vi "FPGA_PPG_VI_Tree.vi"   [LabVIEW 2014, in "NI-FPGA_PPG_Driver.lvlib"]
doc: "This is a VI tree containing all VIs that are available to the user.\n\nDietrich Beck, GSI Helmholtzzentrum fuer Schwerionenforschung, Germany\noriginal author: Falk Ziegler, Falk Ziegler, ziegler@physik.uni-greifswald.de"
uses:
  NI-FPGA_PPG_Driver.lvlib
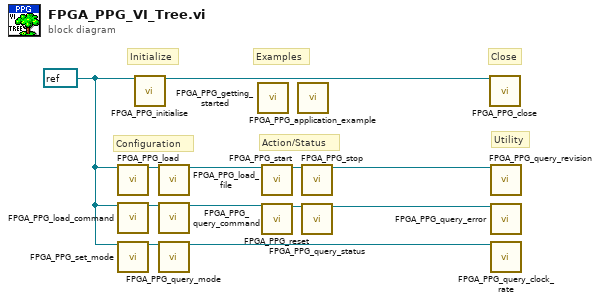
[diagram p0: block diagram]
diagram:
  w8 = refnum<visa-resource-name> refnum ("resource_in")
  # "Examples"
  # "Action/Status"
  # "Configuration"
  # "Utility"
  # "Close"
  # "Initialize"
  n1 = call "FPGA_PPG_load.vi"("resource_in"=w8) -> ("resource_out"=w12:refnum<visa-resource-name>)  [unwired: 17 in, 1 out]
  n2 = call "FPGA_PPG_load_command.vi"("resource_in"=w8) -> ("resource_out"=w3:refnum<visa-resource-name>)  [unwired: 17 in, 1 out]
  n3 = call "FPGA_PPG_set_mode.vi"("resource_in"=w8) -> ("resource_out"=w11:refnum<visa-resource-name>)  [unwired: 17 in, 1 out]
  n4 = call "FPGA_PPG_initialise.vi"("resource_in"=w8) -> ("resource_out"=w10:refnum<visa-resource-name>)  [unwired: 16 in, 2 out]
  n5 = call "FPGA_PPG_load_file.vi"("resource_in"=w12) -> ("resource_out"=w7:refnum<visa-resource-name>)  [unwired: 17 in, 1 out]
  n6 = call "FPGA_PPG_query_command.vi"("resource_in"=w3) -> ("resource_out"=w2:refnum<visa-resource-name>)  [unwired: 16 in, 2 out]
  n7 = call "FPGA_PPG_query_mode.vi"("resource_in"=w11) -> ("resource_out"=w1:refnum<visa-resource-name>)  [unwired: 16 in, 2 out]
  n8 = call "FPGA_PPG_getting_started.vi"() -> ()  [unwired: 1 in]
  n9 = call "FPGA_PPG_start.vi"("resource_in"=w7) -> ("resource_out"=w9:refnum<visa-resource-name>)  [unwired: 17 in, 1 out]
  n10 = call "FPGA_PPG_reset.vi"("resource_in"=w2) -> ("resource_out"=w5:refnum<visa-resource-name>)  [unwired: 17 in, 1 out]
  n11 = call "FPGA_PPG_application_example.vi"() -> ()  [unwired: 1 in]
  n12 = call "FPGA_PPG_stop.vi"("resource_in"=w9) -> ("resource_out"=w6:refnum<visa-resource-name>)  [unwired: 16 in, 2 out]
  n13 = call "FPGA_PPG_query_status.vi"("resource_in"=w5) -> ("resource_out"=w4:refnum<visa-resource-name>)  [unwired: 16 in, 2 out]
  n14 = call "FPGA_PPG_close.vi"("resource_in"=w10) -> ()  [unwired: 18 in, 1 out]
  n15 = call "FPGA_PPG_query_revision.vi"("resource_in"=w6) -> ()  [unwired: 16 in, 3 out]
  n16 = call "FPGA_PPG_query_error.vi"("resource_in"=w4) -> ()  [unwired: 17 in, 2 out]
  n17 = call "FPGA_PPG_query_clock_rate.vi"("resource_in"=w1) -> ()  [unwired: 16 in, 3 out]
